vi "DRWM模块.vi"(1 "通量名称":string[](array[string]), 2 "因子说明":string, 3 "P2名称":string[](array[string]), 5 "SSF因子":cluster{"x":dbl, "y":dbl}[][](array[cluster]), 7 "因子棒名":string[](array[string]), 9 "时间步长":sgl, 10 "反应性in":dbl[](array[numeric]), 11 "通量in":dbl[](array[numeric]), 12 "执行:调用时显示前面板":bool, 14 "P2信号":dbl[](array[numeric])) -> (0 "通量out":dbl[](array[numeric]), 4 "上下段通量索引":u16[](array[numeric]), 6 "DRWM开":bool, 8 "P2信号out":dbl[](array[numeric]), 13 "棒限":dbl[](array[numeric]), 15 "动态棒位":dbl)   [LabVIEW 2020]
uses:
  <vilib>/Analysis/baseanly.llb/Mean (DBL).vi
  <vilib>/Analysis/NI_AALBase.lvlib
panel:
  in  "DSF2合1":bool
  in  "上下段比值":dbl=0.0001 min=0.0001 max=100.0 step=0.0001 format="%0.2f"
  in  "修正因子选择":u16(ring)
  out "修正因子文件说明":string
  in  "底部棒位(步)":dbl=5.0
  in  "触发准备":bool
  out "触发量稳定值":dbl
  in  "反应性触发选择":u16(ring) items=["电流1a", "电流2a"]
  out "触发量散度%":dbl
  in  "触发量容限%":dbl=10.0
  in  "反应性暂存":dbl[](array[numeric])
  in  "棒位暂存":dbl[](array[numeric])
  in  "触发方式":u16(ring)=3 items=["手动触发启动", "反应性触发启动", "棒位触发启动", "实时棒位无需触发"]
  in  "顶部棒位(步)":dbl=225.0
  out "面板开":bool
  in  "棒速(步/分钟)":dbl=72.0
  out "DRWM控制棒":dbl(slide) min=0.0 max=225.0 scale=0.0..225.0
  in  "DRWM启动":bool
  in  "上部探测器选择":u16(ring) items=["电流1a", "电流2a"]
  in  "下部探测器选择":u16(ring)=1 items=["电流1a", "电流2a"]
  in  "控制棒选择":i32(ring) items=["D棒位", "C棒位"]
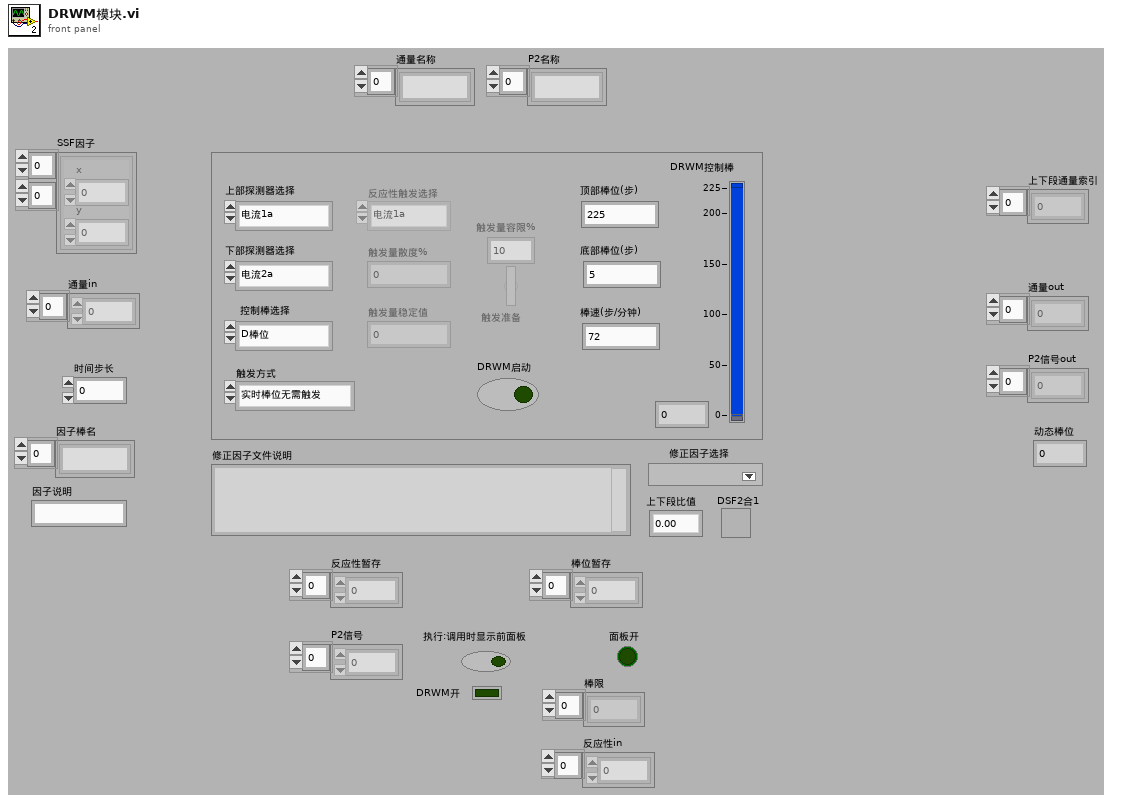
[diagram p1: front panel]
types:
  T1 = enum8{"Enabled", "Disabled", "Disabled and Grayed Out"}
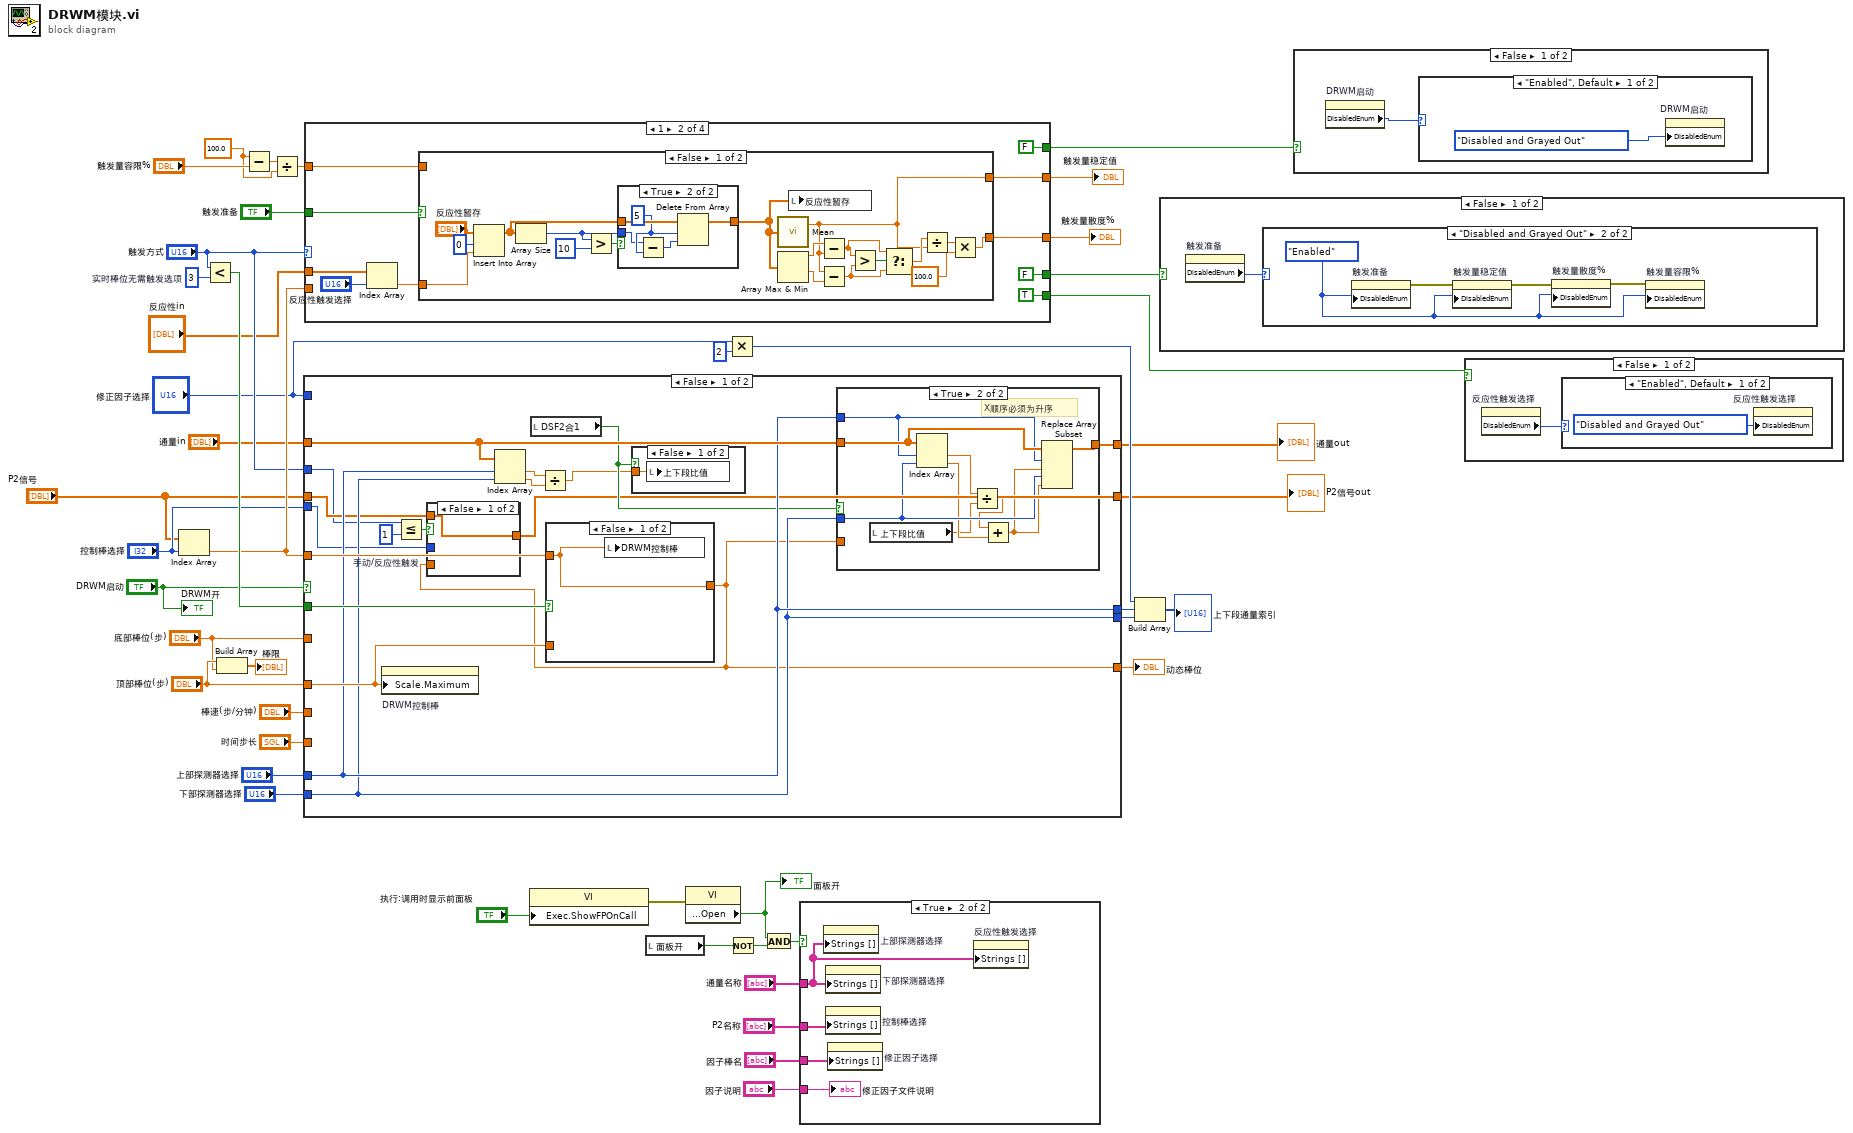
[diagram p0: block diagram]
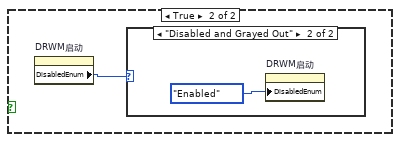
[diagram p3: hidden frame]
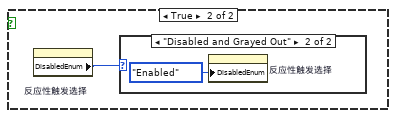
[diagram p6: hidden frame]
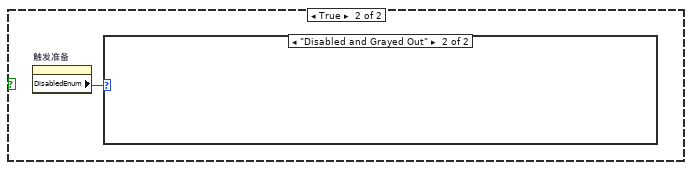
[diagram p9: hidden frame]
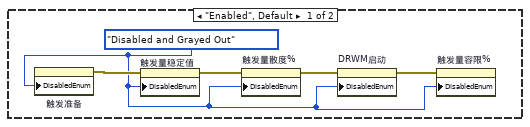
[diagram p10: hidden frame]
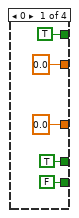
[diagram p11: hidden frame]
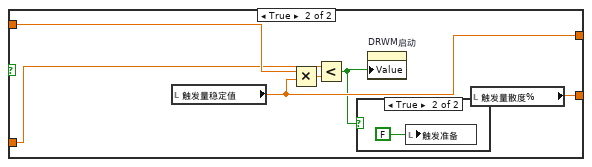
[diagram p13: hidden frame]
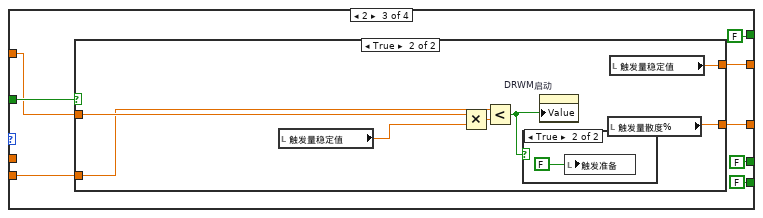
[diagram p15: hidden frame]
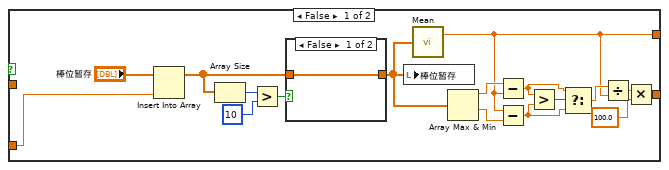
[diagram p16: hidden frame]
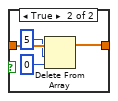
[diagram p17: hidden frame]
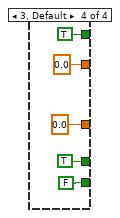
[diagram p19: hidden frame]
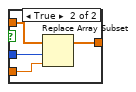
[diagram p20: hidden frame]
diagram:
  w31 = 100.0 ("x")
  w35 = u16 3  # 实时棒位无需触发选项
  n1 = Index Array(array="P2信号", index="控制棒选择") -> (element=w30:dbl)
  n2 = Less?(x="触发方式", y=w35) -> (x < y?=w36:bool)
  n3 = Build Array("顶部棒位(步)", "底部棒位(步)") -> (→"棒限":dbl[])
  n4 = Subtract(x=w31, y="触发量容限%") -> (x-y=w32:dbl)
  n5 = Divide(x=w32, y=w31) -> (x/y=w29:dbl)
  n6 = case shown="False" "DRWM启动" {
    tunnel: "通量in" -> [w58 w107]
    tunnel: [w57 w106] -> w2
    tunnel: "棒速(步/分钟)" -> [_ w102]
    tunnel: "时间步长" -> [_ w98]
    tunnel: "顶部棒位(步)" -> [w61 _]
    tunnel: w36 -> [w62 w100]
    tunnel: w30 -> [w63 w99]
    tunnel: [w56 w84] -> w14
    tunnel: [w55 w83] -> w13
    tunnel: [w50 w82] -> w27
    tunnel: "P2信号" -> [w49 w92]
    tunnel: [w48 w91] -> w4
    tunnel: "触发方式" -> [w47 w95]
    tunnel: "控制棒选择" -> [w51 w90]
    tunnel: "底部棒位(步)" -> [_ w89]
    tunnel: "修正因子选择" -> [_ w88]
    tunnel: "上部探测器选择" -> [w56 w84]
    tunnel: "下部探测器选择" -> [w55 w83]
    frame False {
      w53 = u16 1  # 手动/反应性触发
      n7 = property on="DRWM控制棒" class="Slide (strict)"("Scale.Maximum"=w61) -> ()  [unwired: 2 in, 2 out]
      n8 = Less Or Equal?(x=w47, y=w53) -> (x <= y?=w52:bool)
      n9 = Index Array(array=w58, index #1=w56, index #2=w55) -> (element #1=w60:dbl, element #2=w59:dbl)
      n10 = local read "DSF2合1"() -> (w54:bool)
      n11 = Divide(x=w60, y=w59) -> (x/y=w46:dbl)
      n12 = case shown="False" w62 {
        tunnel: [w80 w81] -> w50
        tunnel: w63 -> [w80 _]
        tunnel: w61 -> [_ w81]
        frame False {
          n13 = local write "DRWM控制棒"(w80) -> ()
        }
        frame True {
          n14 = local write "DRWM控制棒"(w81) -> ()
        }
      }
      n15 = case shown="False" w52 {
        tunnel: w49 -> [w64 w68]
        tunnel: [w64 w67] -> w48
        tunnel: w50 -> [_ w66]
        tunnel: w51 -> [_ w65]
        frame False {
        }
        frame True {
          n16 = Replace Array Subset(array=w68, new element=w66, index=w65) -> (w67:dbl[])
        }
      }
      n17 = case shown="False" w54 {
        tunnel: w46 -> [w79 _]
        frame False {
          n18 = local write "上下段比值"(w79) -> ()
        }
        frame True {
        }
      }
      n19 = case shown="True" w54 {
        tunnel: w58 -> [w69 w78]
        tunnel: [w69 w77] -> w57
        tunnel: w50 -> [_ _]
        tunnel: w56 -> [_ w76]
        tunnel: w55 -> [_ w75]
        frame False {
        }
        frame True {
          # "X顺序必须为升序"
          n20 = local read "上下段比值"() -> (w71:dbl)
          n21 = Index Array(array=w78, index #1=w76, index #2=w75) -> (element #1=w72:dbl, element #2=w73:dbl)
          n22 = Divide(x=w72, y=w71) -> (x/y=w70:dbl)
          n23 = Add(x=w70, y=w73) -> (x+y=w74:dbl)
          n24 = Replace Array Subset(array=w78, new element #1=w74, index #1=w76, new element #2=w74, index #2=w75) -> (w77:dbl[])
        }
      }
    }
    frame True {
      w94 = u16 1  # 手动/反应性触发
      n25 = Divide(x=w102, y=60.0) -> (x/y=w97:dbl)
      n26 = Less Or Equal?(x=w95, y=w94) -> (x <= y?=w93:bool)
      n27 = Multiply(x=w88, y=u16 2) -> (x*y=w85:u16)
      n28 = Multiply(x=w97, y=w98) -> (x*y=w96:dbl)
      n29 = case shown="True" w100 {
        tunnel: w99 -> [w137 _]
        tunnel: [w137 w140] -> w82
        tunnel: w96 -> [_ w145]
        tunnel: w89 -> [w139 w142]
        tunnel: [w138 w141] -> _
        frame False {
          n30 = Greater?(x=w137, y=w139) -> (0:w138:bool)
        }
        frame True {
          n31 = local read "DRWM控制棒"() -> (w143:dbl)
          n32 = Subtract(x=w143, y=w145) -> (x-y=w144:dbl)
          n33 = Greater?(x=w144, y=w142) -> (0:w141:bool)
          n34 = Select(t=w144, s=w141, f=w142) -> (s? t:f=w140:dbl)
        }
      }
      "DRWM控制棒" <- w82
      n35 = case shown="True" w93 {
        tunnel: w92 -> [w132 w136]
        tunnel: [w132 w135] -> w91
        tunnel: w82 -> [_ w134]
        tunnel: w90 -> [_ w133]
        frame False {
        }
        frame True {
          n36 = Replace Array Subset(array=w136, new element=w134, index=w133) -> (w135:dbl[])
        }
      }
      n37 = Increment(x=w85) -> (x+1=w86:u16)
      n38 = Index Array(array="SSF因子", index (row) #1=w85, index (row) #2=w86) -> (element #1=w104:cluster{"x":dbl, "y":dbl}[], element #2=w103:cluster{"x":dbl, "y":dbl}[])  [unwired: 2 in]
      n39 = flat-sequence {
        tunnel: w107 -> [w124]
        tunnel: [w123] -> w106
        tunnel: w104 -> [w122]
        tunnel: w103 -> [w121]
        tunnel: w84 -> [w120]
        tunnel: w83 -> [w119]
        tunnel: w82 -> [w118]
        frame #0 {
          # "X顺序必须为升序"
          n40 = Interpolate 1D Array(1:w118, 2:w122) -> (0:w116:dbl)
          n41 = Interpolate 1D Array(1:w118, 2:w121) -> (0:w115:dbl)
          n42 = Index Array(array=w124, index #1=w120, index #2=w119) -> (element #1=w117:dbl, element #2=w114:dbl)
          n43 = Divide(x=w114, y=w115) -> (x/y=w112:dbl)
          n44 = Divide(x=w117, y=w116) -> (x/y=w113:dbl)
          n45 = case shown="True" "DSF2合1" {
            tunnel: w113 -> [w126 w131]
            tunnel: w112 -> [w125 w129]
            tunnel: [w125 w127] -> w111
            tunnel: [w126 w127] -> w110
            tunnel: "上下段比值" -> [_ w130]
            frame False {
            }
            frame True {
              n46 = Divide(x=w131, y=w130) -> (x/y=w128:dbl)
              n47 = Add(x=w128, y=w129) -> (x+y=w127:dbl)
            }
          }
          n48 = Replace Array Subset(array=w124, new element #1=w110, index #1=w120, new element #2=w111, index #2=w119) -> (w123:dbl[])
        }
      }
    }
  }
  "通量out" <- w2
  "动态棒位" <- w27
  "P2信号out" <- w4
  n49 = case shown="1" "触发方式" {
    tunnel: w30 -> [_ _ w199 _]
    tunnel: w29 -> [_ w154 w196 _]
    tunnel: "反应性in" -> [_ w156 _ _]
    tunnel: [0.0 ("触发量散度%") w160 w198 0.0] -> w28
    tunnel: [0.0 ("mean") w159 w195 0.0 ("触发量稳定值")] -> w26
    tunnel: "触发准备" -> [_ w155 w197 _]
    tunnel: [TRUE FALSE FALSE TRUE] -> w24
    tunnel: [FALSE TRUE FALSE FALSE] -> w23
    tunnel: [TRUE FALSE FALSE TRUE] -> w22
    frame 0 {
    }
    frame 1 {
      n50 = Index Array(array=w156, index="反应性触发选择") -> (element=w157:dbl)
      n51 = case shown="False" w155 {
        tunnel: [w163 w190] -> w160
        tunnel: [w162 w188] -> w159
        tunnel: w157 -> [w161 w185]
        tunnel: w154 -> [_ w186]
        frame False {
          n52 = Insert Into Array(array="反应性暂存", index=0 ("索引"), new element=w161) -> (w175:dbl[])
          n53 = Array Size(array=w175) -> (size(s)=w173:i32)
          n54 = Greater?(x=w173, y=10) -> (0:w178:bool)
          n55 = case shown="True" w178 {
            tunnel: w175 -> [w179 w183]
            tunnel: [w179 w184] -> w174
            tunnel: w173 -> [_ w181]
            frame False {
            }
            frame True {
              w182 = 5 ("长度")
              n56 = Subtract(x=w181, y=w182) -> (x-y=w180:i32)
              n57 = Delete From Array(array=w183, length=w182, index=w180) -> (array with subset deleted=w184:dbl[])  [unwired: 1 out]
            }
          }
          n58 = call-poly <vilib>:"Mean.vi"("X"=w174) -> ("mean"=w162:dbl)  [unwired: 1 out]
          n59 = Array Max & Min(array=w174) -> (max value=w171:dbl, min value=w170:dbl)  [unwired: 2 out]
          n60 = local write "反应性暂存"(w174) -> ()
          n61 = Subtract(x=w171, y=w162) -> (x-y=w168:dbl)
          n62 = Subtract(x=w162, y=w170) -> (x-y=w167:dbl)
          n63 = Greater?(x=w168, y=w167) -> (0:w169:bool)
          n64 = Select(t=w168, s=w169, f=w167) -> (s? t:f=w166:dbl)
          n65 = Divide(x=w166, y=w162) -> (x/y=w165:dbl)
          n66 = Multiply(x=w165, y=100.0) -> (x*y=w163:dbl)
        }
        frame True {
          n67 = local read "触发量稳定值"() -> (w188:dbl)
          n68 = Multiply(x=w186, y=w188) -> (x*y=w189:dbl)
          n69 = Less?(x=w185, y=w189) -> (x < y?=w187:bool)
          n70 = case shown="True" w187 {
            frame False {
            }
            frame True {
              n71 = local write "触发准备"(FALSE ("触发准备")) -> ()
            }
          }
          n72 = property on="DRWM启动" class="Bool (strict)"("Value"=w187) -> ()  [unwired: 2 in, 2 out]
          n73 = local read "触发量散度%"() -> (w190:dbl)
        }
      }
    }
    frame 2 {
      n74 = case shown="True" w197 {
        tunnel: w199 -> [w211 w222]
        tunnel: [w201 w227] -> w198
        tunnel: w196 -> [_ w225]
        tunnel: [w200 w223] -> w195
        frame False {
          n75 = Insert Into Array(array="棒位暂存", new element=w211) -> (w215:dbl[])  [unwired: 1 in]
          n76 = Array Size(array=w215) -> (size(s)=w213:i32)
          n77 = Greater?(x=w213, y=10) -> (0:w216:bool)
          n78 = case shown="False" w216 {
            tunnel: w215 -> [w217 w220]
            tunnel: [w217 w221] -> w207
            frame False {
            }
            frame True {
              n79 = Delete From Array(array=w220, length=5 ("长度"), index=0 ("索引")) -> (array with subset deleted=w221:dbl[])  [unwired: 1 out]
            }
          }
          n80 = local write "棒位暂存"(w207) -> ()
          n81 = call-poly <vilib>:"Mean.vi"("X"=w207) -> ("mean"=w200:dbl)  [unwired: 1 out]
          n82 = Array Max & Min(array=w207) -> (max value=w206:dbl, min value=w210:dbl)  [unwired: 2 out]
          n83 = Subtract(x=w206, y=w200) -> (x-y=w205:dbl)
          n84 = Subtract(x=w200, y=w210) -> (x-y=w208:dbl)
          n85 = Greater?(x=w205, y=w208) -> (0:w209:bool)
          n86 = Select(t=w205, s=w209, f=w208) -> (s? t:f=w202:dbl)
          n87 = Divide(x=w202, y=w200) -> (x/y=w204:dbl)
          n88 = Multiply(x=w204, y=100.0) -> (x*y=w201:dbl)
        }
        frame True {
          n89 = local read "触发量稳定值"() -> (w226:dbl)
          n90 = Multiply(x=w225, y=w226) -> (x*y=w228:dbl)
          n91 = Less?(x=w222, y=w228) -> (x < y?=w224:bool)
          n92 = case shown="True" w224 {
            frame False {
            }
            frame True {
              n93 = local write "触发准备"(FALSE ("触发准备")) -> ()
            }
          }
          n94 = property on="DRWM启动" class="Bool (strict)"("Value"=w224) -> ()  [unwired: 2 in, 2 out]
          n95 = local read "触发量散度%"() -> (w227:dbl)
          n96 = local read "触发量稳定值"() -> (w223:dbl)
        }
      }
    }
    frame 3, Default {
    }
  }
  "触发量散度%" <- w28
  "触发量稳定值" <- w26
  n97 = property class="VI"("Exec.ShowFPOnCall"="执行:调用时显示前面板") -> (error out=w44:errorcluster)  [unwired: 2 in, 1 out]
  n98 = local read "面板开"() -> (w43:bool)
  n99 = property class="VI"(error in=w44) -> ("Front Panel.Open"=w41:bool)  [unwired: 1 in, 2 out]
  "面板开" <- w41
  n100 = Multiply(x="修正因子选择", y=u16 2) -> (x*y=w6:u16)
  n101 = Not(x=w43) -> (.not. x?=w42:bool)
  n102 = And(x=w41, y=w42) -> (x .and. y?=w40:bool)
  n103 = case shown="True" w40 {
    tunnel: "P2名称" -> [_ w238]
    tunnel: "通量名称" -> [_ w237]
    tunnel: "因子棒名" -> [_ w235]
    tunnel: "因子说明" -> [_ w236]
    frame False {
    }
    frame True {
      n104 = property on="上部探测器选择" class="Ring (strict)"("Strings []"=w237) -> ()  [unwired: 2 in, 2 out]
      n105 = property on="下部探测器选择" class="Ring (strict)"("Strings []"=w237) -> ()  [unwired: 2 in, 2 out]
      n106 = property on="控制棒选择" class="Ring (strict)"("Strings []"=w238) -> ()  [unwired: 2 in, 2 out]
      n107 = property on="修正因子选择" class="Ring (strict)"("Strings []"=w235) -> ()  [unwired: 2 in, 2 out]
      n108 = property on="反应性触发选择" class="Ring (strict)"("Strings []"=w237) -> ()  [unwired: 2 in, 2 out]
      "修正因子文件说明" <- w236
    }
  }
  n109 = Build Array(w6, w14, w13) -> (→"上下段通量索引":u16[])
  n110 = case shown="False" w24 {
    frame False {
      n111 = property on="触发准备" class="Bool (strict)"() -> ("DisabledEnum"=w239:T1)  [unwired: 2 in, 2 out]
      n112 = case shown="\"Disabled and Grayed Out\"" w239 {
        frame "Enabled", Default {
        }
        frame "Disabled and Grayed Out" {
          w241 = T1."Enabled" ("禁用")
          n113 = property on="触发准备" class="Bool (strict)"("DisabledEnum"=w241) -> (error out=w243:errorcluster)  [unwired: 2 in, 1 out]
          n114 = property on="触发量稳定值" class="DigNum (strict)"(error in=w243, "DisabledEnum"=w241) -> (error out=w242:errorcluster)  [unwired: 1 in, 1 out]
          n115 = property on="触发量散度%" class="DigNum (strict)"(error in=w242, "DisabledEnum"=w241) -> (error out=w240:errorcluster)  [unwired: 1 in, 1 out]
          n116 = property on="触发量容限%" class="DigNum (strict)"(error in=w240, "DisabledEnum"=w241) -> ()  [unwired: 1 in, 2 out]
        }
      }
    }
    frame True {
      n117 = property on="触发准备" class="Bool (strict)"() -> ("DisabledEnum"=w244:T1)  [unwired: 2 in, 2 out]
      n118 = case shown="\"Disabled and Grayed Out\"" w244 {
        frame "Enabled", Default {
          w245 = T1."Disabled and Grayed Out" ("禁用")
          n119 = property on="触发准备" class="Bool (strict)"("DisabledEnum"=w245) -> (error out=w248:errorcluster)  [unwired: 2 in, 1 out]
          n120 = property on="触发量稳定值" class="DigNum (strict)"(error in=w248, "DisabledEnum"=w245) -> (error out=w249:errorcluster)  [unwired: 1 in, 1 out]
          n121 = property on="触发量散度%" class="DigNum (strict)"(error in=w249, "DisabledEnum"=w245) -> (error out=w247:errorcluster)  [unwired: 1 in, 1 out]
          n122 = property on="DRWM启动" class="Bool (strict)"(error in=w247, "DisabledEnum"=w245) -> (error out=w246:errorcluster)  [unwired: 1 in, 1 out]
          n123 = property on="触发量容限%" class="DigNum (strict)"(error in=w246, "DisabledEnum"=w245) -> ()  [unwired: 1 in, 2 out]
        }
        frame "Disabled and Grayed Out" {
        }
      }
    }
  }
  n124 = case shown="False" w22 {
    frame False {
      n125 = property on="DRWM启动" class="Bool (strict)"() -> ("DisabledEnum"=w250:T1)  [unwired: 2 in, 2 out]
      n126 = case shown="\"Enabled\", Default" w250 {
        frame "Enabled", Default {
          n127 = property on="DRWM启动" class="Bool (strict)"("DisabledEnum"=T1."Disabled and Grayed Out" ("禁用")) -> ()  [unwired: 2 in, 2 out]
        }
        frame "Disabled and Grayed Out" {
        }
      }
    }
    frame True {
      n128 = property on="DRWM启动" class="Bool (strict)"() -> ("DisabledEnum"=w252:T1)  [unwired: 2 in, 2 out]
      n129 = case shown="\"Disabled and Grayed Out\"" w252 {
        frame "Enabled", Default {
        }
        frame "Disabled and Grayed Out" {
          n130 = property on="DRWM启动" class="Bool (strict)"("DisabledEnum"=T1."Enabled" ("禁用")) -> ()  [unwired: 2 in, 2 out]
        }
      }
    }
  }
  n131 = case shown="False" w23 {
    frame False {
      n132 = property on="反应性触发选择" class="Ring (strict)"() -> ("DisabledEnum"=w254:T1)  [unwired: 2 in, 2 out]
      n133 = case shown="\"Enabled\", Default" w254 {
        frame "Enabled", Default {
          n134 = property on="反应性触发选择" class="Ring (strict)"("DisabledEnum"=T1."Disabled and Grayed Out" ("禁用")) -> ()  [unwired: 2 in, 2 out]
        }
        frame "Disabled and Grayed Out" {
        }
      }
    }
    frame True {
      n135 = property on="反应性触发选择" class="Ring (strict)"() -> ("DisabledEnum"=w256:T1)  [unwired: 2 in, 2 out]
      n136 = case shown="\"Disabled and Grayed Out\"" w256 {
        frame "Enabled", Default {
        }
        frame "Disabled and Grayed Out" {
          n137 = property on="反应性触发选择" class="Ring (strict)"("DisabledEnum"=T1."Enabled" ("禁用")) -> ()  [unwired: 2 in, 2 out]
        }
      }
    }
  }
  "DRWM开" <- "DRWM启动"
